vi "Abort Sequence.vi"(8 "error in":errorcluster, 11 "NMR in":refnum<class "NMR.lvclass">) -> (0 "error out":errorcluster, 1 "Stop?":bool, 3 "NMR out":refnum<class "NMR.lvclass">)   [LabVIEW 2011]
uses:
  Modules/Hardware/NMR/NMR.lvclass
  Functional Globals/General Flags.ctl
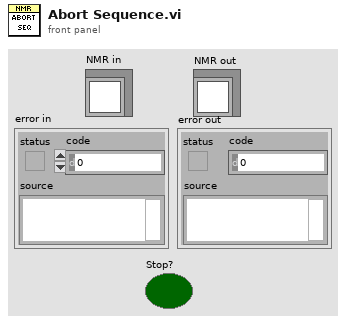
[diagram p1: front panel]
types:
  T1 = typedef "General Flags.ctl" = enum16{"Initialize", "Set Abort Flag", "Get Abort Flag"}
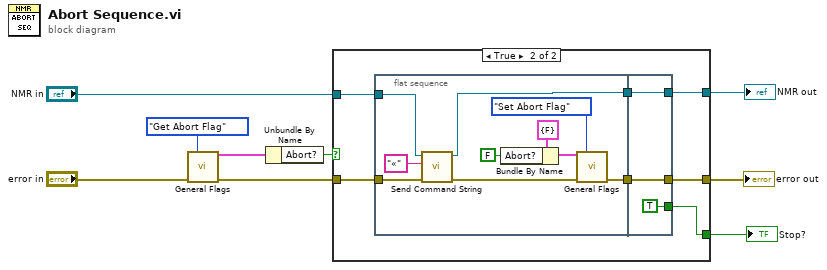
[diagram p0: block diagram]
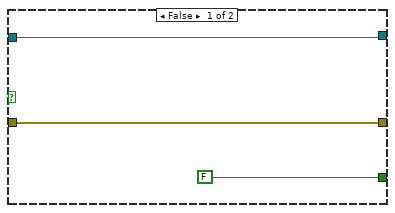
[diagram p2: hidden frame]
diagram:
  n1 = call "General Flags.vi"("action"=General_Flags."Get Abort Flag" ("Action"), "error in"="error in") -> ("General Flags Out"=w7:cluster{"Abort?":bool}, "error out"=w4:errorcluster)  [unwired: 12 in]
  n2 = Unbundle By Name(w7) -> ("Abort?"=w6:bool)
  n3 = case shown="True" w6 {
    tunnel: "NMR in" -> [w11 w19]
    tunnel: w4 -> [w12 w18]
    tunnel: [w12 w16] -> w1
    tunnel: [w11 w17] -> w3
    tunnel: [FALSE w13] -> w2
    frame False {
    }
    frame True {
      n4 = flat-sequence {
        tunnel: w19 -> [w29]
        tunnel: w18 -> [w27]
        tunnel: [w26] -> w15
        tunnel: [w24] -> w14
        tunnel: [w31] -> w16
        tunnel: [w32] -> w17
        tunnel: w15 -> [w32]
        tunnel: w14 -> [w31]
        tunnel: [TRUE] -> w13
        frame #0 {
          n5 = call-dynamic "Send Command String.vi"("error in (no error)"=w27, "Command String"="«", "NMR in"=w29) -> ("error out"=w25:errorcluster, "NMR out"=w26:refnum<class "NMR.lvclass">)  [unwired: 7 in]
          n6 = Bundle By Name(cluster=cluster{"Abort?":bool} {"Abort?"=FALSE} ("General Flags Out"), "Abort?"=FALSE) -> (w21:cluster{"Abort?":bool})
          n7 = call "General Flags.vi"("General Flags In"=w21, "action"=General_Flags."Set Abort Flag" ("Action"), "error in"=w25) -> ("error out"=w24:errorcluster)  [unwired: 11 in, 1 out]
        }
        frame #1 {
        }
      }
    }
  }
  "NMR out" <- w3
  "Stop?" <- w2
  "error out" <- w1
